vi "CRYSet Property in Graph.vi"(10 "Flatten Data String":string, 11 "pGraph VI":refnum<vi>) -> (3 "pGraph VI Out":refnum<vi>)   [LabVIEW 2013]
uses:
  Control/CRYResult Property.ctl
  Control/CRYTable Property.ctl
  Control/CRYPicture Property.ctl
  Control/CRYPolar Property.ctl
  Control/CRYIntensity Property.ctl
  Control/CRYText Property.ctl
panel:
  in  "Text Format":T1
  in  "Intensity Property":T2={"Time Steps"=0, "Frequency Bins"=0, "Type"=0, "Length"=0, "Map Type"=enum."rainbow"} {"Type" items=["Rectangle"=0, "Hanning"=1, "Hamming"=2, "Blackman-Harris"=3, "Exact Blackman"=4, "Blackman"=5, "Flat Top"=6, "4 Term B-Harris"=7, "7 Term B-Harris"=8, "Low Sidelobe"=9, "Blackman Nuttall"=11, "Triangle"=30, "Bartlett-Hanning"=31, "Bohman"=32, "Parzen"=33, "Welch"=34, "Kaiser"=60, "Dolph-Chebyshev"=61, "Gaussian"=62]}
  in  "Polar Property":T3={"polar attributes"={"maximum"=2.0, "minimum"=0.0, "clip to min"=FALSE, "log"=FALSE, "grid color"=3381657, "plot color"=16711680, "fmt and prec"={"format"=enum."Decimal", "precision"=2}, "visible section"=4}, "Auto/Manual"=0, "Zero Adjust (deg)"=0, "Angle Increment (deg)"=0, "Mirror"=FALSE, "Auto Increment"=FALSE, "Total Rotatin (deg)"=0, "Discrete/Rannge"=0, "Show Name"=FALSE, "CurValues"=[], "CurIndex"=0, "CurColors"=[], "CurColors_Range"=[], "CurValues_Range"=[], "Pen"={"Width"=1, "Style"=enum."Solid"}, "BackgroundColor"=0} {"polar attributes"."minimum" format="%0.2f"; "polar attributes"."maximum" format="%0.2f"}
  in  "Picture Property":T4
  in  "Table Property":T5 {"Precision" items=["Digits of precision", "Significant digits"]}
  in  "Result Property":T6={"Show Limits"=FALSE, "Show Yield"=FALSE, "Pass/Fail"=FALSE, "Notation"=0, "Digits"=0, "Precision"=0, "Hide Traling Zeros"=FALSE, "Show vertical scroll bar"=FALSE, "Show horizontal scroll bar"=FALSE, "True"="NO ELECTRICAL SIGNAL DETECTED!\nCheck wiring and connections.", "False"="NO ELECTRICAL SIGNAL DETECTED!\nCheck wiring and connections.", "Font Size"=0, "Overall/Optional"=0} {"Precision" items=["Digits of precision", "Significant digits"]}
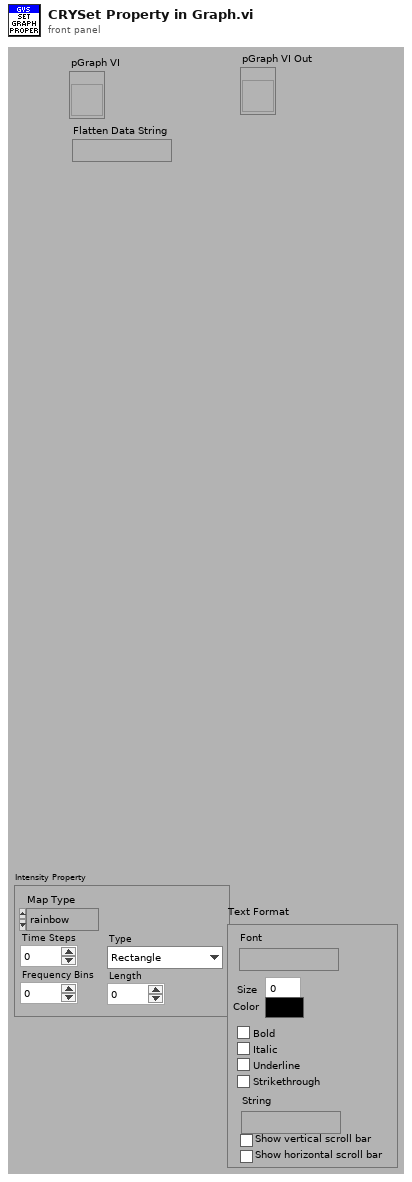
[diagram p1: front panel]
types:
  T1 = typedef "CRYText Property.ctl" = cluster{"Size":u32, "Bold":bool, "Italic":bool, "Underline":bool, "Strikethrough":bool, "Color":u32, "Font":string, "String":string, "Show vertical scroll bar":bool, "Show horizontal scroll bar":bool}
  T2 = typedef "CRYIntensity Property.ctl" = cluster{"Time Steps":i32, "Frequency Bins":i32, "Type":u32, "Length":i32, "Map Type":enum16{"fire", "rainbow", "grey", "inverse grey", "ice", "original"}}
  T3 = typedef "CRYPolar Property.ctl" = cluster{"polar attributes":cluster{"maximum":dbl, "minimum":dbl, "clip to min":bool, "log":bool, "grid color":u32, "plot color":u32, "fmt and prec":cluster{"format":enum8{"Decimal", "Scientific", "Engineering", "Binary", "Octal", "Hex"}, "precision":u8}, "visible section":u16}, "Auto/Manual":u16, "Zero Adjust (deg)":i32, "Angle Increment (deg)":i32, "Mirror":bool, "Auto Increment":bool, "Total Rotatin (deg)":i32, "Discrete/Rannge":u16, "Show Name":bool, "CurValues":dbl[], "CurIndex":u16, "CurColors":u32[], "CurColors_Range":u32[], "CurValues_Range":dbl[], "Pen":cluster{"Width":u16, "Style":enum32{"Solid", "Dash", "Dot", "DashDot", "DashDotDot"}}, "BackgroundColor":u32}
  T4 = typedef "CRYPicture Property.ctl" = cluster{"Image Path":string, "Show vertical scroll bar":bool, "Show horizontal scroll bar":bool}
  T5 = typedef "CRYTable Property.ctl" = cluster{"Reset All Columns":bool, "Transpose":bool, "Display Units":bool, "Notation":u16, "Digits":u16, "Precision":u16, "Hide Traling Zeros":bool, "Column Width":u16, "Row Header Width":u16, "Show vertical scroll bar":bool, "Show horizontal scroll bar":bool}
  T6 = typedef "CRYResult Property.ctl" = cluster{"Show Limits":bool, "Show Yield":bool, "Pass/Fail":bool, "Notation":u16, "Digits":u16, "Precision":u16, "Hide Traling Zeros":bool, "Show vertical scroll bar":bool, "Show horizontal scroll bar":bool, "True":string, "False":string, "Font Size":u16, "Overall/Optional":u16}
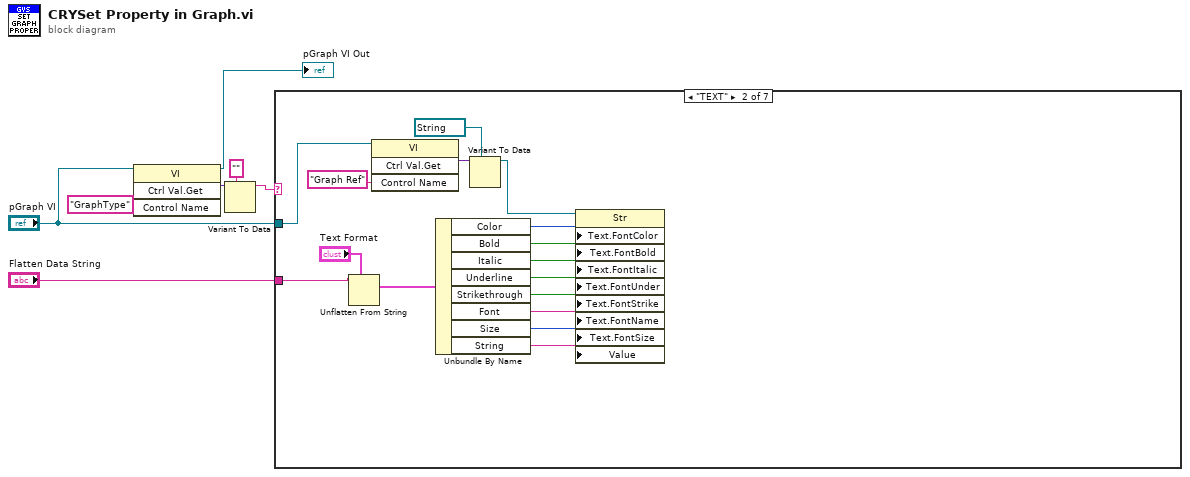
[diagram p0: block diagram]
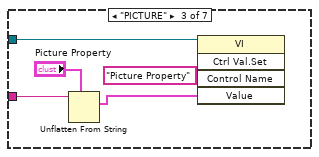
[diagram p3: hidden frame]
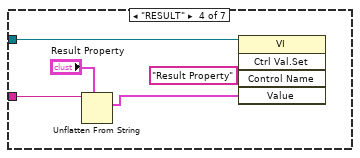
[diagram p4: hidden frame]
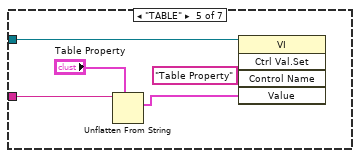
[diagram p5: hidden frame]
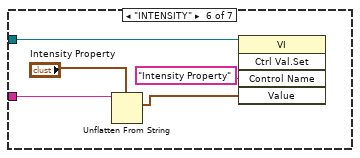
[diagram p6: hidden frame]
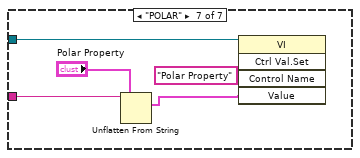
[diagram p7: hidden frame]
diagram:
  n1 = invoke class="VI" method="Ctrl Val.Get"(reference="pGraph VI", "Control Name"="GraphType") -> (reference out=→"pGraph VI Out":refnum<vi>, "Get Control Value Variant"=w6:variant)  [unwired: 2 in, 2 out]
  n2 = Variant To Data(type="" ("Control Name"), Variant=w6) -> (data=w4:string)  [unwired: 1 in, 1 out]
  n3 = case shown="\"TEXT\"" w4 {
    tunnel: "Flatten Data String" -> [_ w23 w26 w30 w36 w41 w46]
    tunnel: "pGraph VI" -> [_ w19 w27 w32 w37 w42 w47]
    frame Default {
    }
    frame "TEXT" {
      n4 = Unflatten From String(type="Text Format", binary string=w23) -> (value=w10:T1)  [unwired: 1 in, 4 out]
      n5 = invoke class="VI" method="Ctrl Val.Get"(reference=w19, "Control Name"="Graph Ref") -> ("Get Control Value Variant"=w21:variant)  [unwired: 2 in, 3 out]
      n6 = Unbundle By Name(w10) -> ("Color"=w11:u32, "Bold"=w12:bool, "Italic"=w13:bool, "Underline"=w14:bool, "Strikethrough"=w15:bool, "Font"=w16:string, "Size"=w17:u32, "String"=w18:string)
      n7 = Variant To Data(type=refnum<vi> refnum ("Graph Ref"), Variant=w21) -> (data=w9:refnum<vi>)  [unwired: 1 in, 1 out]
      n8 = property class="Str"(reference=w9, "Text.FontColor"=w11, "Text.FontBold"=w12, "Text.FontItalic"=w13, "Text.FontUnder"=w14, "Text.FontStrike"=w15, "Text.FontName"=w16, "Text.FontSize"=w17, "Value"=w18) -> ()  [unwired: 1 in, 2 out]
    }
    frame "PICTURE" {
      n9 = Unflatten From String(type="Picture Property", binary string=w26) -> (value=w24:T4)  [unwired: 1 in, 4 out]
      n10 = invoke class="VI" method="Ctrl Val.Set"(reference=w27, "Control Name"="Picture Property", "Value"=w24) -> ()  [unwired: 2 in, 5 out]
    }
    frame "RESULT" {
      n11 = Unflatten From String(type="Result Property", binary string=w30) -> (value=w29:T6)  [unwired: 1 in, 4 out]
      n12 = invoke class="VI" method="Ctrl Val.Set"(reference=w32, "Control Name"="Result Property", "Value"=w29) -> ()  [unwired: 2 in, 5 out]
    }
    frame "TABLE" {
      n13 = Unflatten From String(type="Table Property", binary string=w36) -> (value=w34:T5)  [unwired: 1 in, 4 out]
      n14 = invoke class="VI" method="Ctrl Val.Set"(reference=w37, "Control Name"="Table Property", "Value"=w34) -> ()  [unwired: 2 in, 5 out]
    }
    frame "INTENSITY" {
      n15 = Unflatten From String(type="Intensity Property", binary string=w41) -> (value=w39:T2)  [unwired: 1 in, 4 out]
      n16 = invoke class="VI" method="Ctrl Val.Set"(reference=w42, "Control Name"="Intensity Property", "Value"=w39) -> ()  [unwired: 2 in, 5 out]
    }
    frame "POLAR" {
      n17 = Unflatten From String(type="Polar Property", binary string=w46) -> (value=w44:T3)  [unwired: 1 in, 4 out]
      n18 = invoke class="VI" method="Ctrl Val.Set"(reference=w47, "Control Name"="Polar Property", "Value"=w44) -> ()  [unwired: 2 in, 5 out]
    }
  }
